vi "GetActual.vi"(5 "error in (no error)":errorcluster) -> (16 "Actual":T1, 19 "error out":errorcluster)   [LabVIEW 2014, in "IndoorData.lvclass"]
uses:
  IndoorData.lvclass
  ActualValues.ctl
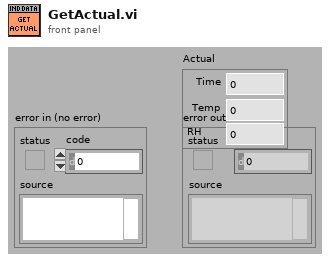
[diagram p1: front panel]
types:
  T1 = typedef "IndoorData.lvclass/ActualValues.ctl" = cluster{"Time":dbl, "Temp":dbl, "RH":dbl}
  T2 = typedef "IndoorData.lvclass/ObjectAttributes.ctl" = cluster{"DebugData":T3, "Actual":T1}
  T3 = typedef "IndoorData.lvclass/DebugData.ctl" = cluster{"Rev":string, "Location":string, "LoopIdx":i32, "PiCoreTemp":dbl, "Error":errorcluster}
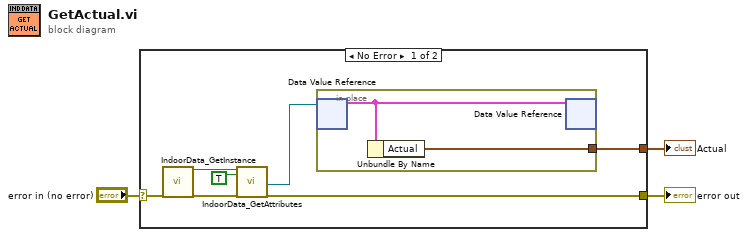
[diagram p0: block diagram]
diagram:
  n1 = case shown="No Error" "error in (no error)" {
    selector: "error in (no error)" -> [w8 w13]
    tunnel: [w10 w13] -> w2
    tunnel: [w4 _] -> w1
    frame No Error {
      n2 = call "IndoorData_GetInstance.vi"("error in (no error)"=w8) -> ("reference out"=w9:refnum<class "IndoorData.lvclass">, "error out"=w7:errorcluster)  [unwired: 14 in, 3 out]
      n3 = call "IndoorData_GetAttributes.vi"("reference in"=w9, "OnlyGetDvrReference(False)"=TRUE, "error in (no error)"=w7) -> ("DataRef"=w6:refnum<data-value>, "error out"=w10:errorcluster)  [unwired: 13 in, 2 out]
      n4 = in-place {
        in-place-border: [w12] -> w4
        n5 = in-place-dvr #1(w6) -> (w11:T2)  [unwired: 1 out]
        n6 = Unbundle By Name(w11) -> ("Actual"=w12:T1)
        n7 = in-place-dvr #1(w11) -> ()  [unwired: 2 out]
      }
    }
    frame Error {
    }
  }
  "error out" <- w2
  "Actual" <- w1
